vi "lsl push sample s.vi"(8 "error in (no error)":errorcluster, 10 "data":i16[](array[numeric]), 11 "outlet":T1) -> (0 "error out":errorcluster, 2 "function return":i32)   [LabVIEW 2018, in "liblsl-LabVIEW.lvlib"]
doc: "extern LIBLSL_C_API int32_t lsl_push_sample_s(lsl_outlet out, const int16_t *data);"
uses:
  <userlib>/liblsl-LabVIEW/liblsl-LabVIEW.lvlib
  <userlib>/liblsl-LabVIEW/Custom Controls/lsl_outlet.ctl
  <userlib>/liblsl-LabVIEW/liblsl64.dll
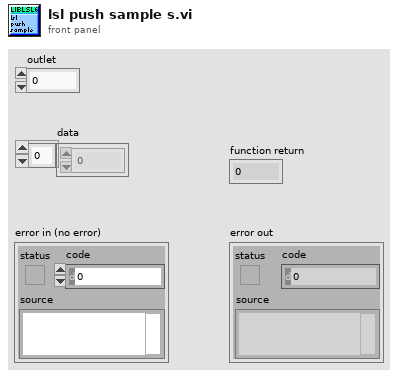
[diagram p1: front panel]
types:
  T1 = typedef "liblsl-LabVIEW.lvlib/lsl_outlet.ctl" = u64
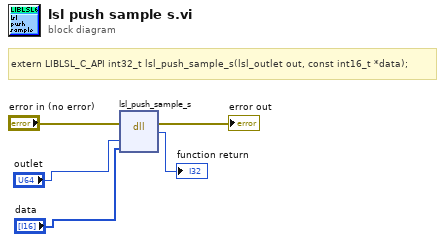
[diagram p0: block diagram]
diagram:
  # "extern LIBLSL_C_API int32_t lsl_push_sample_s(lsl_outlet out, const int16_t *data);"
  n1 = dll-call lib="C:/Program Files/National Instruments/LabVIEW 2018/user.lib/liblsl-LabVIEW/liblsl64.*" fn="lsl_push_sample_s"(error in="error in (no error)", "out"="outlet", "data"="data") -> (error out=→"error out":errorcluster, "return type"=→"function return":i32)  [unwired: 4 in, 1 out]
